vi "Configure Source.vi"(8 "error in (no error)":errorcluster, 10 "Source (F:Volt)":bool, 11 "Manual PSU in":refnum<class "Manual PSU.lvclass">) -> (0 "error out":errorcluster, 3 "Manual PSU out":refnum<class "Manual PSU.lvclass">)   [LabVIEW 2020, in "Manual PSU.lvclass"]
uses:
  Manual PSU.lvclass
  C:/Sandbox/Git_Sandbox/WiSpry Test Framework source code (LV20)/WiSpry Test Framework/Instruments/Power Supply/Power Supply.lvclass
  Controls/Source mode.ctl
  Power Supply.lvclass/Power Supply.ctl
  Power Supply.lvclass
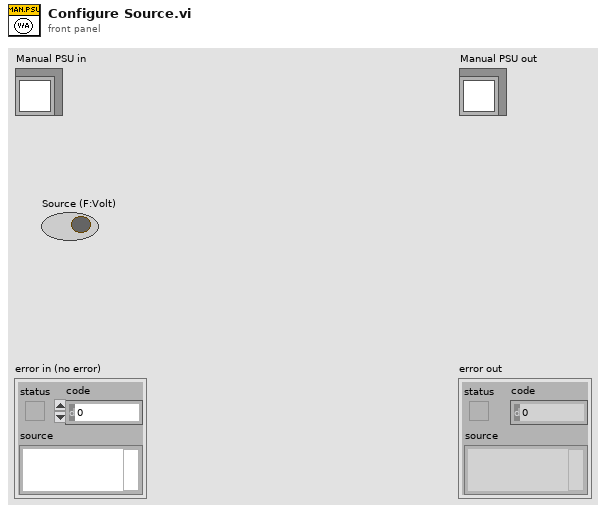
[diagram p1: front panel]
types:
  T1 = typedef "Power Supply.lvclass/Source mode.ctl" = enum32{"Voltage", "Current"}
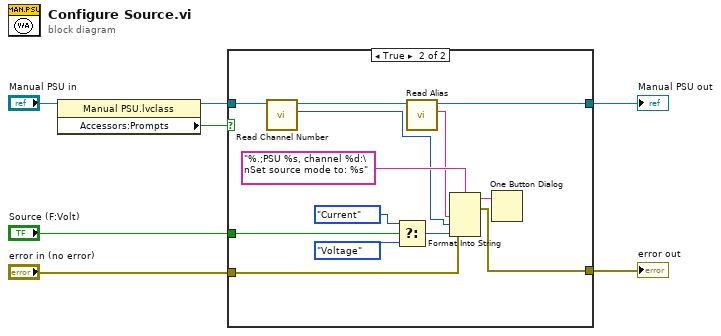
[diagram p0: block diagram]
diagram:
  n1 = property class="Manual PSU.lvclass"(reference="Manual PSU in") -> (reference out=w2:refnum<class "Manual PSU.lvclass">, "Accessors:Prompts"=w1:bool)  [unwired: 1 in, 1 out]
  n2 = case shown="True" w1 {
    tunnel: "error in (no error)" -> [w9 w17]
    tunnel: [w9 w16] -> w6
    tunnel: "Source (F:Volt)" -> [_ w15]
    tunnel: [w8 w13] -> w4
    tunnel: w2 -> [w8 w10]
    frame False {
    }
    frame True {
      n3 = call "Read Channel Number.vi"("Power Supply in"=w10) -> ("Channel Number"=w11:u8, "Power Supply out"=w12:refnum<class "Manual PSU.lvclass">)  [unwired: 9 in]
      n4 = Select(t=Source_mode."Current" ("Source"), s=w15, f=Source_mode."Voltage" ("Source")) -> (s? t:f=w18:T1)
      n5 = call-dynamic "Read Alias.vi"("Power Supply in"=w12) -> ("Alias"=w14:string, "Power Supply out"=w13:refnum<class "Manual PSU.lvclass">)  [unwired: 9 in]
      n6 = Format Into String(format string="%.;PSU %s, channel %d:\nSet source mode to: %s", error in=w17, w14, w11, w18) -> (resulting string=w21:string, error out=w16:errorcluster)  [unwired: 1 in]
      n7 = One Button Dialog(message=w21) -> ()  [unwired: 1 in, 1 out]
    }
  }
  "error out" <- w6
  "Manual PSU out" <- w4
